vi "destroy.vi"(8 "error in":errorcluster, 10 "timeout in ms (-1)":i32=-1, 11 "communicator in":refnum<class "communicator.lvclass">) -> (0 "error out":errorcluster)   [LabVIEW 2015, in "communicator.lvclass"]
uses:
  communicator.lvclass
  communicator.lvclass/communicator.ctl
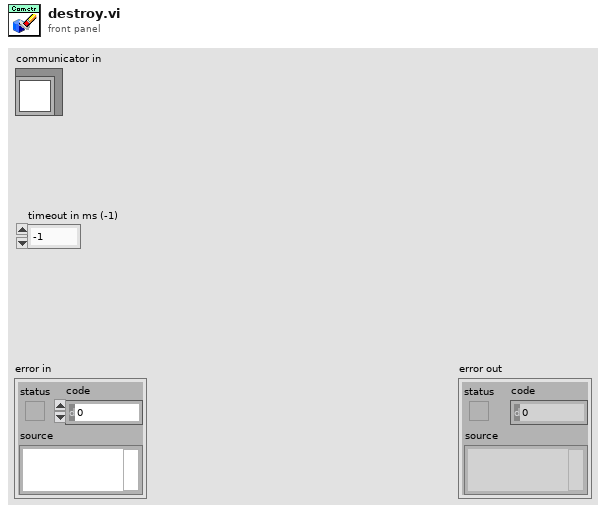
[diagram p1: front panel]
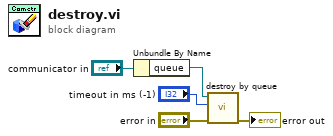
[diagram p0: block diagram]
diagram:
  n1 = Unbundle By Name("communicator in") -> ("queue"=w4:refnum<class "identifying queue.lvclass">)
  n2 = call "destroy by queue.vi"("error in"="error in", "timeout in ms (-1)"="timeout in ms (-1)", "queue"=w4) -> ("error out"=→"error out":errorcluster)  [unwired: 7 in, 1 out]
